vi "Wire Encode Varint I32.vi"(10 "I32":i32, 11 "Buffer in":u8[](array[numeric]) format="%.0x") -> (3 "Buffer":u8[](array[numeric]) format="%.0x")   [LabVIEW 2020, in "LV-Proto.lvlib"]
uses:
  LV-Proto.lvlib
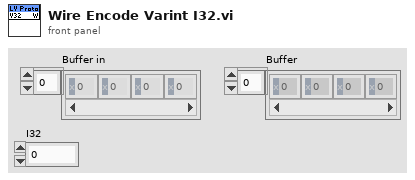
[diagram p1: front panel]
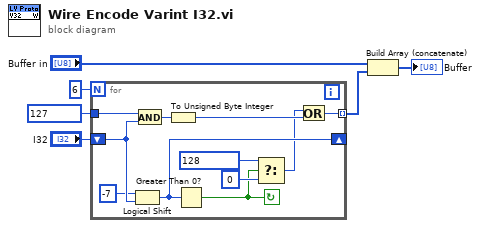
[diagram p0: block diagram]
diagram:
  n1 = for {
    N: 6 -> [_]
    shift-right: [w14] -> _
    shift-left: "I32" -> [w16]
    tunnel: 127 -> [w17]
    tunnel: [w11] -> w1 mode=indexing
    stop <- w8 continue-if-true
    n2 = Logical Shift(y=i16 -7, x=w16) -> (x << y=w14:i32)
    n3 = And(x=w17, y=w16) -> (x .and. y?=w13:i32)
    n4 = To Unsigned Byte Integer(number=w13) -> (unsigned 8bit integer=w12:u8)
    n5 = Greater Than 0?(x=w14) -> (x > 0?=w8:bool)
    n6 = Select(t=u8 128, s=w8, f=u8 0) -> (s? t:f=w7:u8)
    n7 = Or(x=w7, y=w12) -> (x .or. y?=w11:u8)
  }
  n8 = Build Array (concatenate)("Buffer in", w1) -> (→"Buffer":u8[])
